vi "buy robots (1 resource).vi"(7 "cost of X robot":i32, 10 "no. X robots in":i32, 11 "robot's resource in":i32) -> (2 "no. X robots out":i32, 3 "robot's resource out":i32)   [LabVIEW 2019]
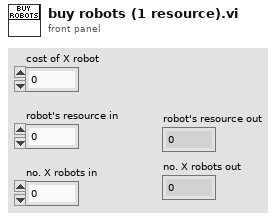
[diagram p1: front panel]
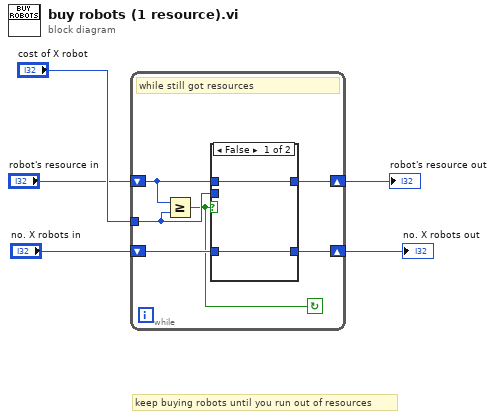
[diagram p0: block diagram]
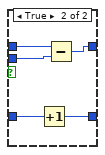
[diagram p2: hidden frame]
diagram:
  # "keep buying robots until you run out of resources"
  n1 = while {
    tunnel: "cost of X robot" -> [w10]
    shift-right: [w11] -> w5
    shift-left: "robot's resource in" -> [w9]
    shift-right: [w8] -> w2
    shift-left: "no. X robots in" -> [w7]
    stop <- w6 continue-if-true
    # "while still got resources"
    n2 = Greater Or Equal?(x=w9, y=w10) -> (x >= y?=w6:bool)
    n3 = case shown="False" w6 {
      tunnel: [w13 w18] -> w8
      tunnel: w7 -> [w13 w17]
      tunnel: w9 -> [w12 w16]
      tunnel: w10 -> [_ w15]
      tunnel: [w12 w14] -> w11
      frame False {
      }
      frame True {
        n4 = Increment(x=w17) -> (x+1=w18:i32)
        n5 = Subtract(x=w16, y=w15) -> (x-y=w14:i32)
      }
    }
  }
  "robot's resource out" <- w5
  "no. X robots out" <- w2
